vi "GetTestResult.vi"(11 "GuiRef":T1) -> (1 "FailStep":string, 2 "PASS/FAIL":bool)   [LabVIEW 2013]
uses:
  Ctl/LEDState.ctl
panel:
  out "FAIL项目":string
  out "PASS项目":string
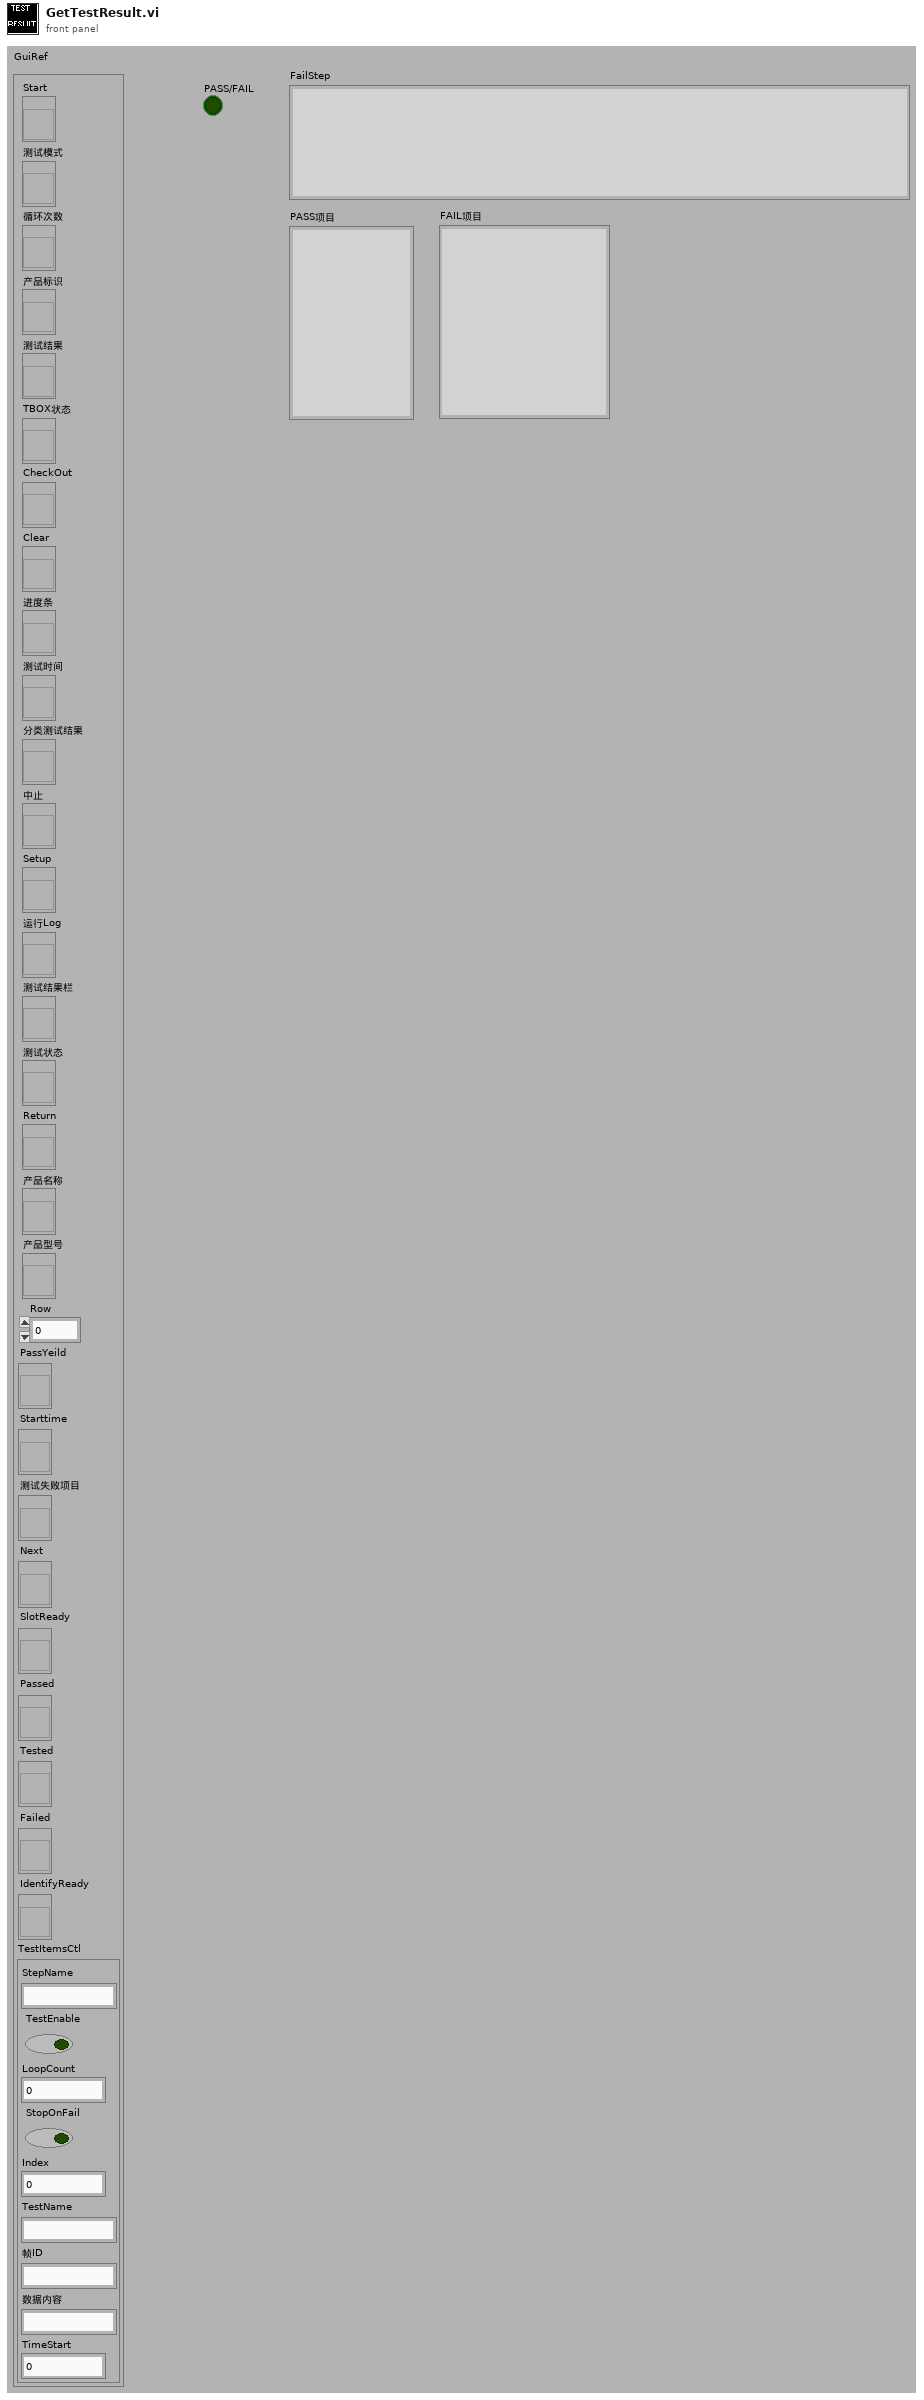
[diagram p1: front panel]
types:
  T1 = typedef "控件.ctl" = cluster{"Start":refnum<vi>, "测试模式":refnum<vi>, "循环次数":refnum<vi>, "产品标识":refnum<vi>, "测试结果":refnum<vi>, "TBOX状态":refnum<vi>, "CheckOut":refnum<vi>, "Clear":refnum<vi>, "进度条":refnum<vi>, "测试时间":refnum<vi>, "分类测试结果":refnum<vi>, "中止":refnum<vi>, "Setup":refnum<vi>, "运行Log":refnum<vi>, "测试结果栏":refnum<vi>, "测试状态":refnum<vi>, "Return":refnum<vi>, "产品名称":refnum<vi>, "产品型号":refnum<vi>, "Row":i32, "PassYeild":refnum<vi>, "Starttime":refnum<vi>, "测试失败项目":refnum<vi>, "Next":refnum<vi>, "SlotReady":refnum<vi>, "Passed":refnum<vi>, "Tested":refnum<vi>, "Failed":refnum<vi>, "IdentifyReady":refnum<vi>, "TestItemsCtl":cluster{"StepName":string, "TestEnable":bool, "LoopCount":u32, "StopOnFail":bool, "Index":u32, "TestName":string, "帧ID":string, "数据内容":string, "TimeStart":u32}}
  T2 = typedef "LEDState.ctl" = enum16{"默认", "闪烁", "停止闪烁", "真", "假"}
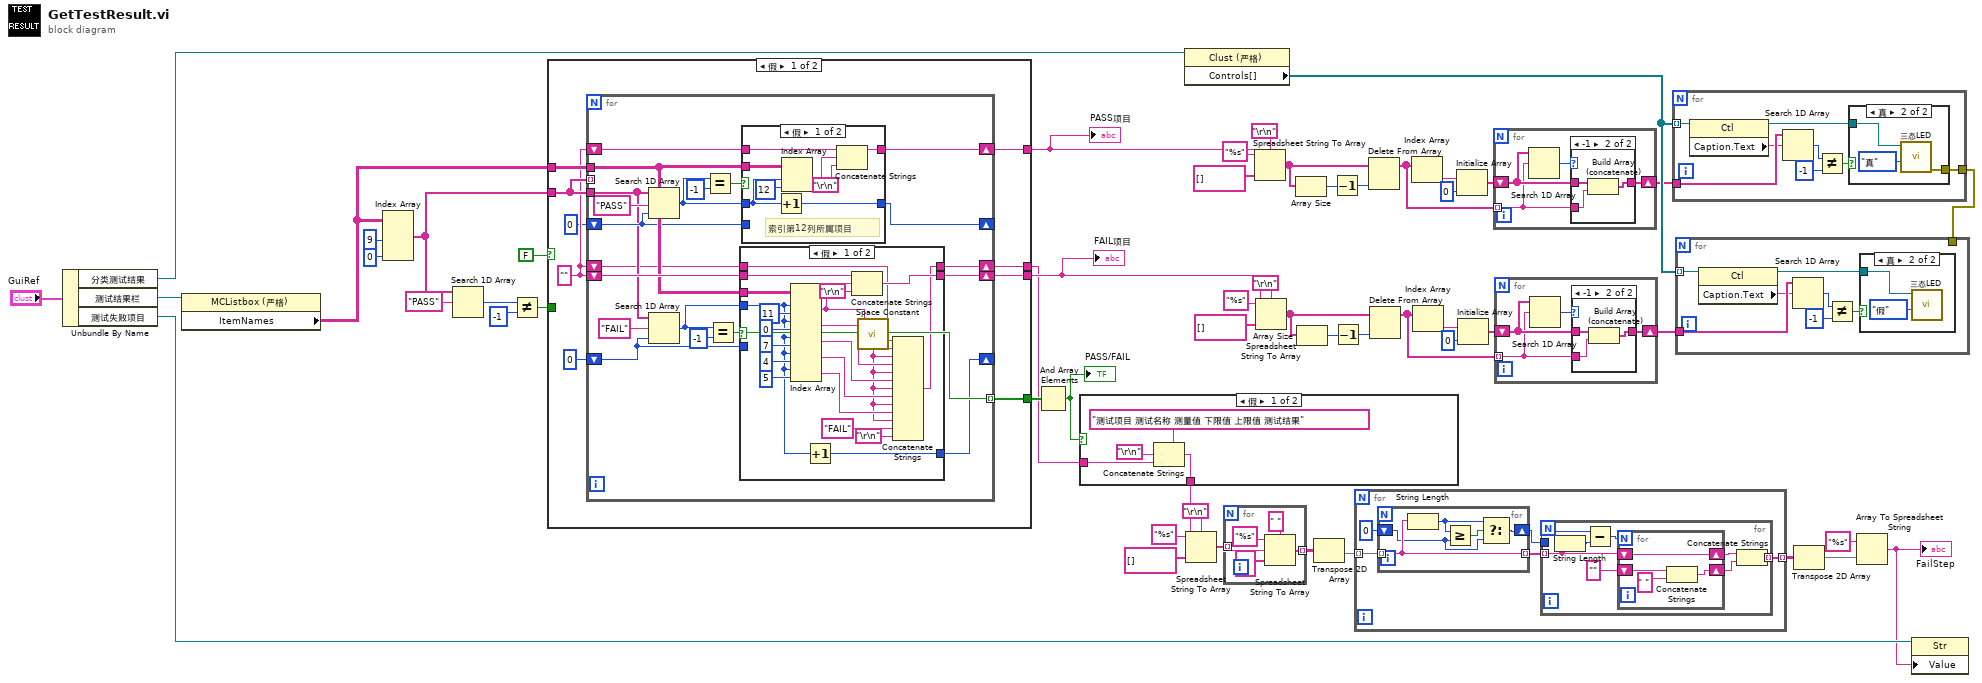
[diagram p0: block diagram]
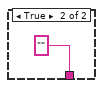
[diagram p2: hidden frame]
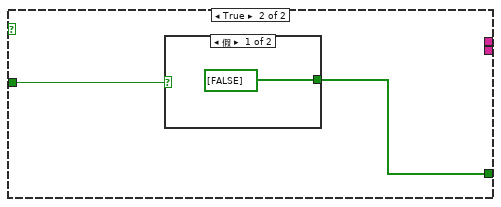
[diagram p9: hidden frame]
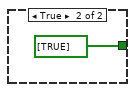
[diagram p10: hidden frame]
diagram:
  n1 = Unbundle By Name("GuiRef") -> ("分类测试结果"=w39:refnum<vi>, "测试结果栏"=w44:refnum<vi>, "测试失败项目"=w15:refnum<vi>)
  n2 = property class="MCListbox (严格)"(reference=w44) -> ("ItemNames"=w43:string[][])  [unwired: 1 in, 2 out]
  n3 = Index Array(array=w43, index (col) #1=9 ("禁用的索引 (列)"), index (col) #2=0 ("index (col)")) -> (element #1=w47:string[])  [unwired: 2 in, 1 out]
  n4 = Search 1D Array(1D array=w47, element="PASS" ("元素")) -> (index of element=w49:i32)  [unwired: 1 out]
  n5 = Not Equal?(x=w49, y=-1) -> (x != y?=w48:bool)
  n6 = case shown="假" FALSE {
    tunnel: w43 -> [w62 _]
    tunnel: w47 -> [w59 _]
    tunnel: [w61 w118] -> w52
    tunnel: [w60 _] -> w16
    tunnel: w48 -> [_ w117]
    tunnel: [w57 _] -> w19
    tunnel: [w55 _] -> w3
    frame False {
      w56 = "" ("字符串")
      n7 = for "For循环" {
        tunnel: w59 -> [w66]
        tunnel: w62 -> [w68]
        tunnel: [w78] -> w61 mode=indexing
        shift-right: [w69] -> w57
        shift-left: w56 -> [w70]
        shift-right: [w80] -> w60
        shift-left: w56 -> [w79]
        shift-right: [w76] -> _
        shift-left: 0 ("y") -> [w75]
        tunnel: w59 -> [_] mode=indexing
        shift-right: [w65] -> _
        shift-left: 0 -> [w67]
        shift-right: [w63] -> w55
        shift-left: w56 -> [w64]
        n8 = Search 1D Array(1D array=w66, element="PASS" ("元素"), start index (0)=w67) -> (index of element=w74:i32)
        n9 = Search 1D Array(1D array=w66, element="FAIL" ("元素"), start index (0)=w75) -> (index of element=w77:i32)
        n10 = Equal?(x=w74, y=-1) -> (x = y?=w73:bool)
        n11 = Equal?(x=w77, y=-1) -> (x = y?=w78:bool)
        n12 = case shown="假" w78 {
          tunnel: w68 -> [w112 _]
          tunnel: [w111 w116] -> w80
          tunnel: w79 -> [w110 w116]
          tunnel: w77 -> [w95 _]
          tunnel: [w109 w115] -> w76
          tunnel: w75 -> [_ w115]
          tunnel: w64 -> [w107 w114]
          tunnel: [w105 w114] -> w63
          frame False {
            n13 = Index Array(array=w112, index (row) #1=w95, index (col) #1=11 ("禁用的索引 (列)"), index (row) #2=w95, index (col) #2=0 ("禁用的索引 (列)"), index (row) #3=w95, index (col) #3=7 ("禁用的索引 (列)"), index (row) #4=w95, index (col) #4=4 ("禁用的索引 (列)"), index (row) #5=w95, index (col) #5=5 ("禁用的索引 (列)")) -> (element #1=w93:string, element #2=w96:string, element #3=w97:string, element #4=w98:string, element #5=w99:string)
            n14 = Increment(x=w95) -> (x+1=w109:i32)
            n15 = Concatenate Strings(w110, w93, "\r\n") -> (w111:string)
            n16 = call <vilib>:"Space Constant.vi"() -> ("String"=w94:string)
            n17 = Concatenate Strings(w107, w93, w94, w96, w94, w97, w94, w98, w94, w99, w94, "FAIL" ("字符串"), "\r\n") -> (w105:string)
          }
          frame True {
          }
        }
        n18 = case shown="假" w73 {
          tunnel: w68 -> [w89 _]
          tunnel: [w88 w92] -> w69
          tunnel: w70 -> [w87 w92]
          tunnel: w74 -> [w84 _]
          tunnel: [w85 w91] -> w65
          tunnel: w67 -> [_ w91]
          frame False {
            # "索引第12列所属项目"
            n19 = Increment(x=w84) -> (x+1=w85:i32)
            n20 = Index Array(array=w89, index (row)=w84, index (col)=12 ("禁用的索引 (列)")) -> (element=w86:string)
            n21 = Concatenate Strings(w87, w86, "\r\n") -> (w88:string)
          }
          frame True {
          }
        }
      }
    }
    frame True {
      n22 = case shown="假" w117 {
        tunnel: [bool[] [FALSE] bool[] [TRUE]] -> w118
        frame False {
        }
        frame True {
        }
      }
    }
  }
  "PASS项目" <- w19
  "FAIL项目" <- w16
  n23 = And Array Elements(Boolean array=w52) -> (logical AND=w2:bool)
  "PASS/FAIL" <- w2
  n24 = case shown="假" w2 {
    tunnel: [w123 ""] -> w4
    tunnel: w3 -> [w122 _]
    frame False {
      n25 = Concatenate Strings("测试项目 测试名称 测量值 下限值 上限值 测试结果" ("字符串"), "\r\n", w122) -> (w123:string)
    }
    frame True {
    }
  }
  n26 = property class="Clust (严格)"(reference=w39) -> ("Controls[]"=w30:refnum<vi>[])  [unwired: 1 in, 2 out]
  n27 = Spreadsheet String To Array(delimiter (Tab)="\r\n", format string="%s" ("格式字符串"), spreadsheet string=w4, array type (2D Dbl)=string[] []) -> (array=w6:string[])
  n28 = for "For循环" {
    tunnel: w6 -> [w128] mode=indexing
    tunnel: [w126] -> w14 mode=indexing
    n29 = Spreadsheet String To Array(delimiter (Tab)=" " ("分隔符(Tab)"), format string="%s" ("格式字符串"), spreadsheet string=w128, array type (2D Dbl)=string[] []) -> (array=w126:string[])
  }
  n30 = Spreadsheet String To Array(delimiter (Tab)="\r\n", format string="%s" ("格式字符串"), spreadsheet string=w19, array type (2D Dbl)=string[] []) -> (array=w29:string[])
  n31 = Spreadsheet String To Array(delimiter (Tab)="\r\n", format string="%s" ("格式字符串"), spreadsheet string=w16, array type (2D Dbl)=string[] []) -> (array=w32:string[])
  n32 = Array Size(array=w29) -> (size(s)=w26:i32)
  n33 = Array Size(array=w32) -> (size(s)=w35:i32)
  n34 = Transpose 2D Array(2D array=w14) -> (transposed array=w13:string[][])
  n35 = Decrement(x=w26) -> (x-1=w27:i32)
  n36 = Decrement(x=w35) -> (x-1=w34:i32)
  n37 = for "For循环" {
    tunnel: w13 -> [w133] mode=indexing
    tunnel: [w132] -> w10 mode=indexing
    n38 = for "For循环" {
      tunnel: w133 -> [w152] mode=indexing
      shift-right: [w148] -> w131
      shift-left: 0 -> [w150]
      tunnel: [w152] -> w134 mode=indexing
      n39 = String Length(string=w152) -> (length=w151:i32)
      n40 = Greater Or Equal?(x=w151, y=w150) -> (x >= y?=w149:bool)
      n41 = Select(t=w151, s=w149, f=w150) -> (s? t:f=w148:i32)
    }
    n42 = for "For循环" {
      tunnel: w134 -> [w136] mode=indexing
      tunnel: [w141] -> w132 mode=indexing
      tunnel: w131 -> [w139]
      n43 = String Length(string=w136) -> (length=w143:i32)
      n44 = Subtract(x=w139, y=w143) -> (x-y=w142:i32)
      n45 = for "For循环" {
        N: w142 -> [_]
        shift-right: [w145] -> w138
        shift-left: "" -> [w146]
        shift-right: [w144] -> w137
        shift-left: w136 -> [w144]
        n46 = Concatenate Strings(w146, " ") -> (w145:string)
      }
      n47 = Concatenate Strings(w137, w138) -> (w141:string)
    }
  }
  n48 = Delete From Array(array=w29, index=w27) -> (array with subset deleted=w28:string[])  [unwired: 1 in, 1 out]
  n49 = Delete From Array(array=w32, index=w34) -> (array with subset deleted=w33:string[])  [unwired: 1 in, 1 out]
  n50 = Index Array(array=w28) -> (element=w23:string)  [unwired: 1 in]
  n51 = Index Array(array=w33) -> (element=w38:string)  [unwired: 1 in]
  n52 = Initialize Array(w23, 0 ("维数大小")) -> (w25:string[])
  n53 = Initialize Array(w38, 0 ("维数大小")) -> (w36:string[])
  n54 = for "For循环" {
    shift-right: [w154] -> w18
    shift-left: w25 -> [w155]
    tunnel: w28 -> [w153] mode=indexing
    n55 = Search 1D Array(1D array=w155, element=w153) -> (index of element=w156:i32)  [unwired: 1 in]
    n56 = case shown="-1" w156 {
      tunnel: w155 -> [w157 w159]
      tunnel: [w157 w158] -> w154
      tunnel: w153 -> [_ w160]
      frame 1, Default {
      }
      frame -1 {
        n57 = Build Array (concatenate)(w159, w160) -> (w158:string[])
      }
    }
  }
  n58 = for "For循环" {
    shift-right: [w162] -> w31
    shift-left: w36 -> [w163]
    tunnel: w33 -> [w161] mode=indexing
    n59 = Search 1D Array(1D array=w163, element=w161) -> (index of element=w164:i32)  [unwired: 1 in]
    n60 = case shown="-1" w164 {
      tunnel: w163 -> [w165 w167]
      tunnel: [w165 w166] -> w162
      tunnel: w161 -> [_ w168]
      frame 1, Default {
      }
      frame -1 {
        n61 = Build Array (concatenate)(w167, w168) -> (w166:string[])
      }
    }
  }
  n62 = for "For循环" {
    tunnel: w30 -> [w176] mode=indexing
    tunnel: w18 -> [w175]
    tunnel: [w169] -> w17
    n63 = property class="Ctl"(reference=w176) -> (reference out=w170:refnum<vi>, "Caption.Text"=w174:string)  [unwired: 1 in, 1 out]
    n64 = Search 1D Array(1D array=w175, element=w174) -> (index of element=w173:i32)  [unwired: 1 in]
    n65 = Not Equal?(x=w173, y=-1) -> (x != y?=w171:bool)
    n66 = case shown="真" w171 {
      tunnel: w170 -> [_ w179]
      tunnel: [_ w177] -> w169
      frame False {
      }
      frame True {
        n67 = call "三态LED.vi"("State"=LEDState."真", "Ctl引用句柄"=w179) -> ("error out"=w177:errorcluster)  [unwired: 4 in, 1 out]
      }
    }
  }
  n68 = for "For循环" {
    tunnel: w30 -> [w186] mode=indexing
    tunnel: w31 -> [w185]
    tunnel: w17 -> [_]
    n69 = property class="Ctl"(reference=w186) -> (reference out=w180:refnum<vi>, "Caption.Text"=w184:string)  [unwired: 1 in, 1 out]
    n70 = Search 1D Array(1D array=w185, element=w184) -> (index of element=w183:i32)  [unwired: 1 in]
    n71 = Not Equal?(x=w183, y=-1) -> (x != y?=w181:bool)
    n72 = case shown="真" w181 {
      tunnel: w180 -> [_ w188]
      frame False {
      }
      frame True {
        n73 = call "三态LED.vi"("State"=LEDState."假", "Ctl引用句柄"=w188) -> ()  [unwired: 4 in, 2 out]
      }
    }
  }
  n74 = Transpose 2D Array(2D array=w10) -> (transposed array=w11:string[][])
  n75 = Array To Spreadsheet String(array=w11, 3:"%s" ("format string")) -> (spreadsheet string=w5:string)  [unwired: 1 out]
  "FailStep" <- w5
  n76 = property class="Str"(reference=w15, "Value"=w5) -> ()  [unwired: 1 in, 2 out]
